vi "Write background.vi"(8 "error in (no error)":errorcluster, 10 "background":dbl[](array[numeric]), 11 "dummyCam in":refnum<class "dummyCam.lvclass">) -> (0 "error out":errorcluster, 3 "dummyCam out":refnum<class "dummyCam.lvclass">)   [LabVIEW 2019, in "dummyCam.lvclass"]
uses:
  dummyCam.lvclass
  _cameraBase/_cameraBase.lvclass
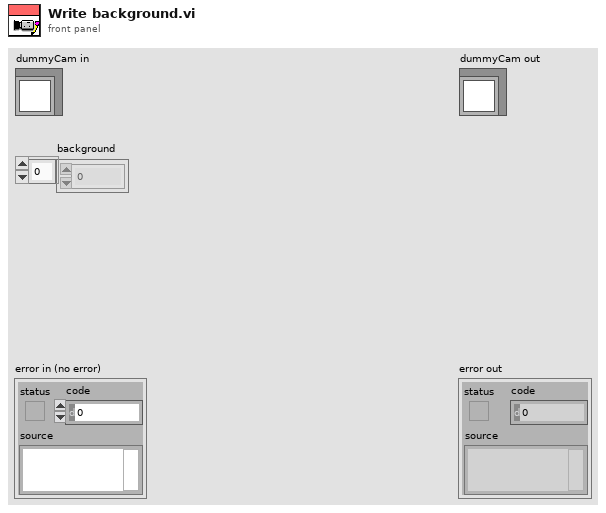
[diagram p1: front panel]
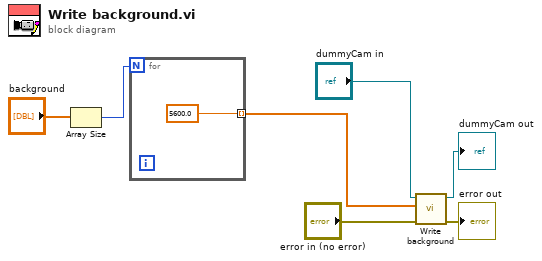
[diagram p0: block diagram]
diagram:
  n1 = Array Size(array="background") -> (size(s)=w2:i32)
  n2 = for {
    N: w2 -> [_]
    tunnel: [5600.0] -> w1 mode=indexing
  }
  n3 = call-parent "Write background.vi"("error in (no error)"="error in (no error)", "background"=w1, "_cameraBase in"="dummyCam in") -> ("error out"=→"error out":errorcluster, "_cameraBase out"=→"dummyCam out":refnum<class "dummyCam.lvclass">)  [unwired: 7 in]
